vi "BRig_RT__Case_Exp__State_WrongOrTimeout_Pre__v4.vi"(0 "input_dataCurrent":u16[](array[numeric]), 5 "input_WorTO":bool, 7 "input_dataBlock":u16[][](array[numeric]), 9 "input_dataTrial":u16[][](array[numeric]), 11 "input_dataExp":u16[](array[numeric])) -> (1 "output_BTPR":bool, 2 "output_T2R":bool, 3 "output_T2R_or_BTPR":u16, 4 "output_dataCurrent":u16[](array[numeric]), 8 "output_dataBlock":u16[][](array[numeric]), 10 "output_dataTrial":u16[][](array[numeric]), 12 "output_BTPRavg":dbl, 13 "output_T2Ravg":dbl, 14 "output_R(F)_or_L(T)":bool, 15 "output_haveNewAvg":bool)   [LabVIEW 2014]
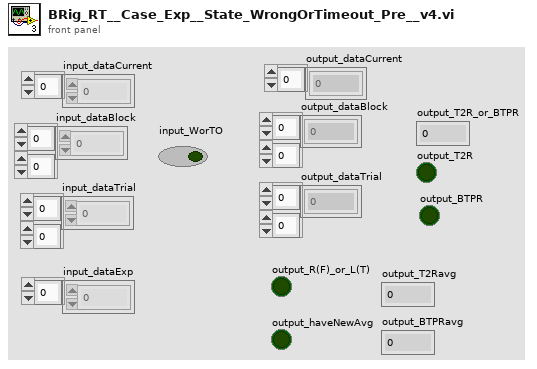
[diagram p1: front panel]
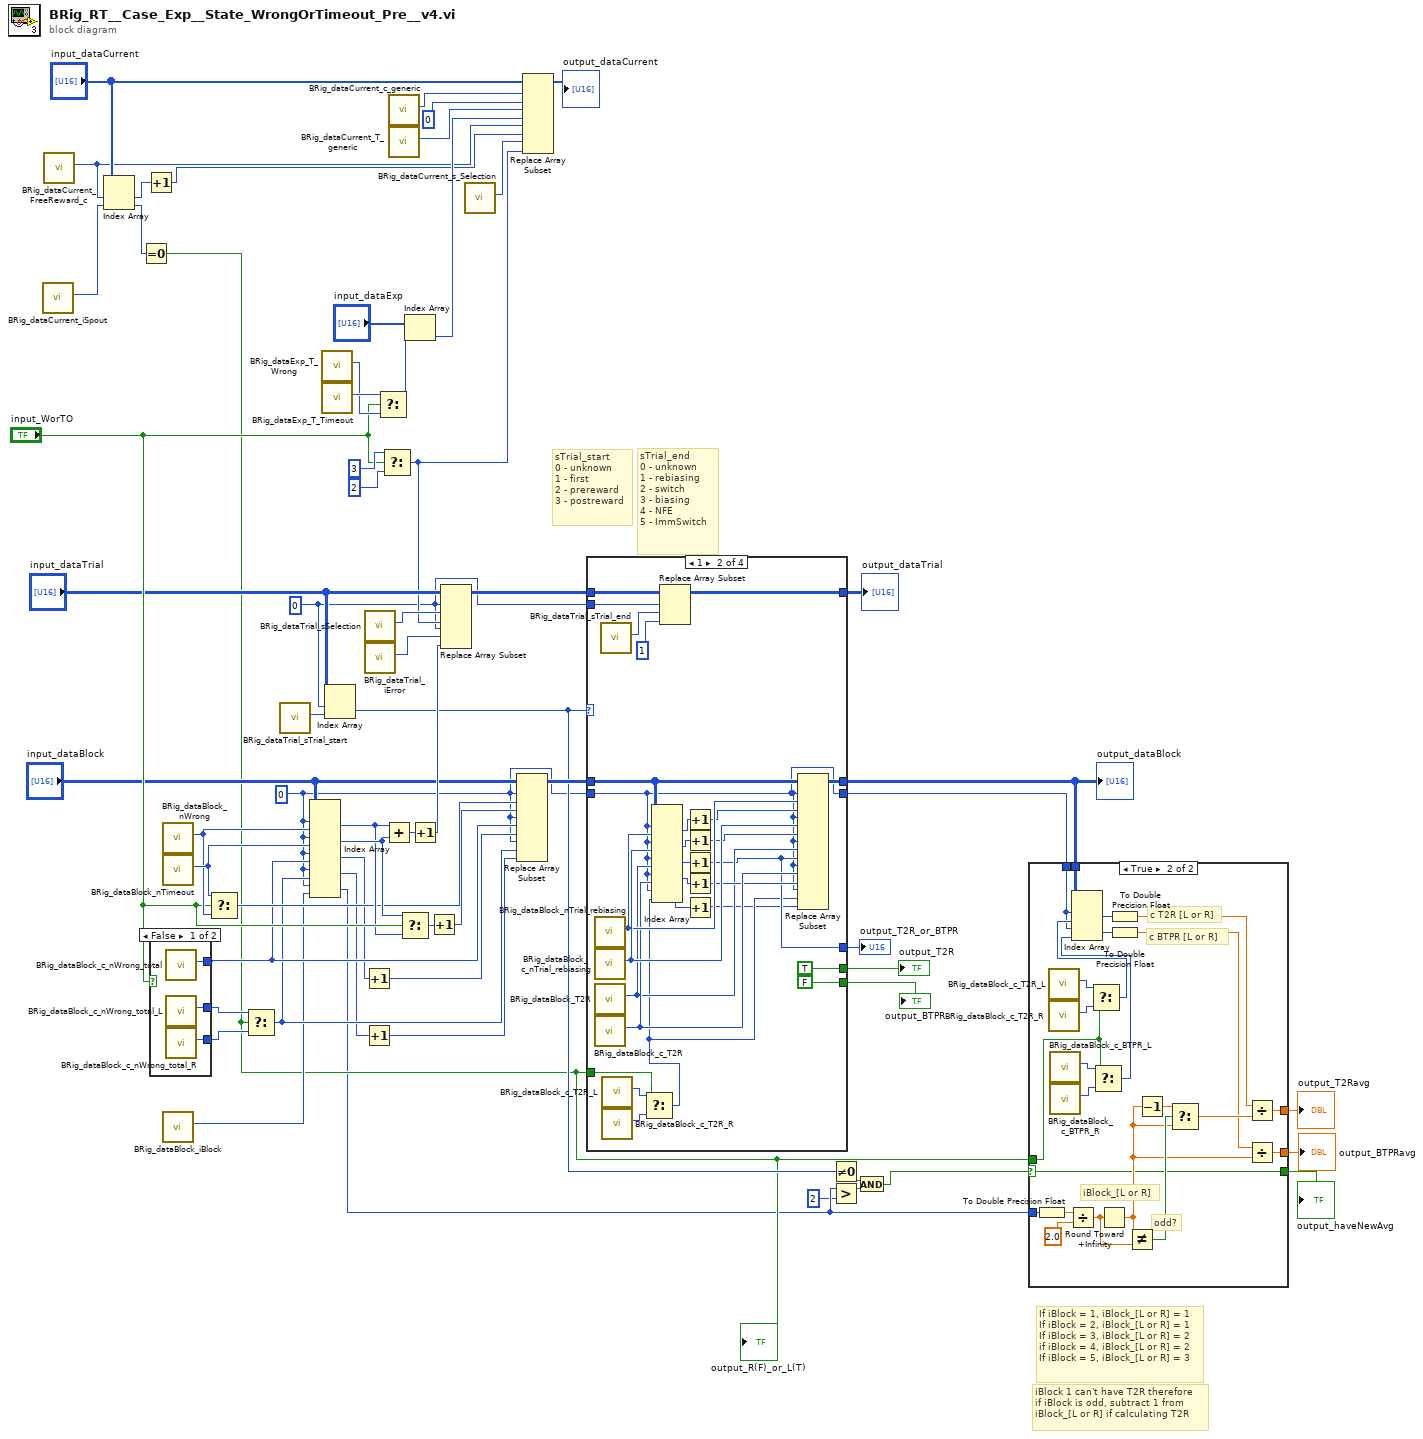
[diagram p0: block diagram]
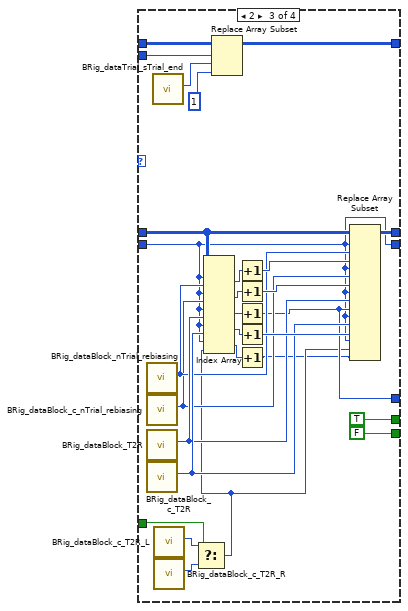
[diagram p4: hidden frame]
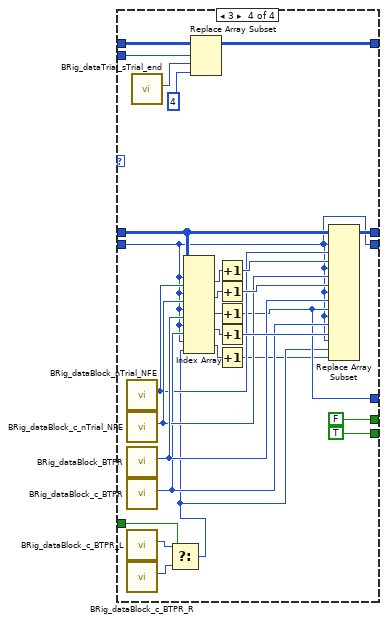
[diagram p5: hidden frame]
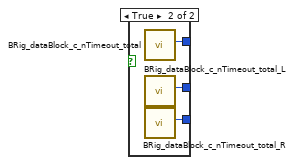
[diagram p6: hidden frame]
diagram:
  w14 = 0
  w15 = 0
  # "iBlock 1 can't have T2R therefore\nif iBlock is odd, subtract 1 from\niBlock_[L or R] if calculating T2R"
  # "If iBlock = 1, iBlock_[L or R] = 1\nIf iBlock = 2, iBlock_[L or R] = 1\nIf iBlock = 3, iBlock_[L or R] = 2\nif iBlock = 4, iBlock_[L or R] = 2\nIf iBlock = 5, iBlock_[L or R] = 3"
  # "sTrial_end\n0 - unknown\n1 - rebiasing\n2 - switch\n3 - biasing\n4 - NFE\n5 - ImmSwitch"
  # "sTrial_start\n0 - unknown\n1 - first\n2 - prereward\n3 - postreward"
  n1 = call "BRig_dataCurrent_iSpout.vi"() -> ("output_iSpout"=w13:i32)  [unwired: 11 in]
  n2 = call "BRig_dataCurrent_FreeReward_c.vi"() -> ("output_FreeReward_c"=w24:i32)  [unwired: 11 in]
  n3 = Index Array(array="input_dataCurrent", index #1=w24, index #2=w13) -> (element #1=w25:u16, element #2=w12:u16)
  n4 = Equal To 0?(x=w12) -> (x = 0?=w11:bool)
  "output_R(F)_or_L(T)" <- w11
  n5 = Increment(x=w25) -> (x+1=w23:u16)
  n6 = case shown="False" "input_WorTO" {
    tunnel: [w66 w69] -> w36
    tunnel: [w65 w68] -> w49
    tunnel: [w64 w67] -> w48
    frame False {
      n7 = call "BRig_dataBlock_c_nWrong_total.vi"() -> ("output_c_nWrong_total"=w66:i32)  [unwired: 11 in]
      n8 = call "BRig_dataBlock_c_nWrong_total_L.vi"() -> ("output_c_nWrong_total_L"=w65:i32)  [unwired: 11 in]
      n9 = call "BRig_dataBlock_c_nWrong_total_R.vi"() -> ("output_c_nWrong_total_R"=w64:i32)  [unwired: 11 in]
    }
    frame True {
      n10 = call "BRig_dataBlock_c_nTimeout_total.vi"() -> ("output_c_nTimeout_total"=w69:i32)  [unwired: 11 in]
      n11 = call "BRig_dataBlock_c_nTimeout_total_L.vi"() -> ("output_c_nTimeout_total_L"=w68:i32)  [unwired: 11 in]
      n12 = call "BRig_dataBlock_c_nTimeout_total_R.vi"() -> ("output_c_nTimeout_total_R"=w67:i32)  [unwired: 11 in]
    }
  }
  n13 = call "BRig_dataBlock_nWrong.vi"() -> ("output_nWrong"=w44:i32)  [unwired: 11 in]
  n14 = call "BRig_dataBlock_nTimeout.vi"() -> ("output_nTimeout"=w45:i32)  [unwired: 11 in]
  n15 = call "BRig_dataBlock_iBlock.vi"() -> ("output_iBlock"=w17:i32)  [unwired: 11 in]
  n16 = Select(t=w45, s="input_WorTO", f=w44) -> (s? t:f=w38:i32)
  n17 = Select(t=w49, s=w11, f=w48) -> (s? t:f=w35:i32)
  n18 = call "BRig_dataTrial_sTrial_start.vi"() -> ("output_sTrial_start"=w30:i32)  [unwired: 11 in]
  n19 = Index Array(array="input_dataBlock", index (row) #1=w14, index (col) #1=w44, index (row) #2=w14, index (col) #2=w45, index (row) #3=w14, index (col) #3=w36, index (row) #4=w14, index (col) #4=w35, index (row) #5=w14, index (col) #5=w17) -> (element #1=w41:u16, element #2=w42:u16, element #3=w34:u16, element #4=w33:u16, element #5=w5:u16)
  n20 = call "BRig_dataExp_T_Wrong.vi"() -> ("output_T_Wrong"=w55:i32)  [unwired: 11 in]
  n21 = call "BRig_dataExp_T_Timeout.vi"() -> ("output_T_Timeout"=w56:i32)  [unwired: 11 in]
  n22 = Index Array(array="input_dataTrial", index (row)=w15, index (col)=w30) -> (element=w16:u16)
  n23 = Increment(x=w34) -> (x+1=w32:u16)
  n24 = Increment(x=w33) -> (x+1=w31:u16)
  n25 = call "BRig_dataTrial_sSelection.vi"() -> ("output_sSelection"=w51:i32)  [unwired: 11 in]
  n26 = call "BRig_dataTrial_iError.vi"() -> ("output_iError"=w50:i32)  [unwired: 11 in]
  n27 = Select(t=w56, s="input_WorTO", f=w55) -> (s? t:f=w57:i32)
  n28 = Select(t=u16 3 ("new element/subarray"), s="input_WorTO", f=u16 2 ("new element/subarray")) -> (s? t:f=w21:u16)
  n29 = Add(x=w41, y=w42) -> (x+y=w47:u16)
  n30 = call "BRig_dataCurrent_c_generic.vi"() -> ("output_count_generic"=w62:i32)  [unwired: 11 in]
  n31 = call "BRig_dataCurrent_T_generic.vi"() -> ("output_T_generic"=w61:i32)  [unwired: 11 in]
  n32 = Select(t=w42, s="input_WorTO", f=w41) -> (s? t:f=w40:u16)
  n33 = Index Array(array="input_dataExp", index=w57) -> (element=w54:u16)
  n34 = Increment(x=w47) -> (x+1=w46:u16)
  n35 = Increment(x=w40) -> (x+1=w37:u16)
  n36 = Replace Array Subset(array="input_dataTrial", new element #1=w21, index (row) #1=w15, index (col) #1=w51, new element #2=w46, index (row) #2=w15, index (col) #2=w50) -> (w28:u16[][])
  n37 = call "BRig_dataCurrent_s_Selection.vi"() -> ("output_s_Selection"=w22:i32)  [unwired: 11 in]
  n38 = Replace Array Subset(array="input_dataBlock", new element #1=w37, index (row) #1=w14, index (col) #1=w38, new element #2=w32, index (row) #2=w14, index (col) #2=w36, new element #3=w31, index (row) #3=w14, index (col) #3=w35) -> (w27:u16[][])
  n39 = Replace Array Subset(array="input_dataCurrent", new element #1=u16 0 ("new element/subarray"), index #1=w62, new element #2=w54, index #2=w61, new element #3=w23, index #3=w24, new element #4=w21, index #4=w22) -> (→"output_dataCurrent":u16[])
  n40 = case shown="1" w16 {
    tunnel: w28 -> [w72 w100 w128 w156]
    tunnel: w15 -> [_ w98 w126 w154]
    tunnel: [w72 w99 w127 w155] -> w26
    tunnel: w27 -> [w71 w89 w112 w144]
    tunnel: [w71 w88 w111 w143] -> w10
    tunnel: w14 -> [w70 w73 w101 w129]
    tunnel: [_ w80 w110 w136] -> w20
    tunnel: [_ TRUE TRUE FALSE] -> w19
    tunnel: [_ FALSE FALSE TRUE] -> w18
    tunnel: w11 -> [_ w79 w103 w135]
    tunnel: [w70 w73 w101 w129] -> w9
    frame 0, Default {
    }
    frame 1 {
      n41 = call "BRig_dataBlock_nTrial_rebiasing.vi"() -> ("output_nTrial_rebiasing"=w94:i32)  [unwired: 11 in]
      n42 = call "BRig_dataBlock_c_nTrial_rebiasing.vi"() -> ("output_c_nTrial_rebiasing"=w95:i32)  [unwired: 11 in]
      n43 = call "BRig_dataBlock_T2R.vi"() -> ("output_T2R"=w83:i32)  [unwired: 11 in]
      n44 = call "BRig_dataBlock_c_T2R.vi"() -> ("output_c_T2R"=w85:i32)  [unwired: 11 in]
      n45 = call "BRig_dataTrial_sTrial_end.vi"() -> ("output_sTrial_end"=w97:i32)  [unwired: 11 in]
      n46 = call "BRig_dataBlock_c_T2R_L.vi"() -> ("output_c_T2R_L"=w78:i32)  [unwired: 11 in]
      n47 = call "BRig_dataBlock_c_T2R_R.vi"() -> ("output_c_T2R_R"=w77:i32)  [unwired: 11 in]
      n48 = Select(t=w78, s=w79, f=w77) -> (s? t:f=w75:i32)
      n49 = Index Array(array=w89, index (row) #1=w73, index (col) #1=w94, index (row) #2=w73, index (col) #2=w95, index (row) #3=w73, index (col) #3=w83, index (row) #4=w73, index (col) #4=w85, index (row) #5=w73, index (col) #5=w75) -> (element #1=w93:u16, element #2=w91:u16, element #3=w87:u16, element #4=w86:u16, element #5=w76:u16)
      n50 = Replace Array Subset(array=w100, new element=u16 1 ("new element/subarray"), index (row)=w98, index (col)=w97) -> (w99:u16[][])
      n51 = Increment(x=w93) -> (x+1=w92:u16)
      n52 = Increment(x=w91) -> (x+1=w90:u16)
      n53 = Increment(x=w87) -> (x+1=w80:u16)
      n54 = Increment(x=w86) -> (x+1=w84:u16)
      n55 = Increment(x=w76) -> (x+1=w74:u16)
      n56 = Replace Array Subset(array=w89, new element #1=w92, index (row) #1=w73, index (col) #1=w94, new element #2=w90, index (row) #2=w73, index (col) #2=w95, new element #3=w80, index (row) #3=w73, index (col) #3=w83, new element #4=w84, index (row) #4=w73, index (col) #4=w85, new element #5=w74, index (row) #5=w73, index (col) #5=w75) -> (w88:u16[][])
    }
    frame 2 {
      n57 = call "BRig_dataBlock_nTrial_rebiasing.vi"() -> ("output_nTrial_rebiasing"=w114:i32)  [unwired: 11 in]
      n58 = call "BRig_dataBlock_c_nTrial_rebiasing.vi"() -> ("output_c_nTrial_rebiasing"=w113:i32)  [unwired: 11 in]
      n59 = call "BRig_dataBlock_T2R.vi"() -> ("output_T2R"=w121:i32)  [unwired: 11 in]
      n60 = call "BRig_dataBlock_c_T2R.vi"() -> ("output_c_T2R"=w122:i32)  [unwired: 11 in]
      n61 = call "BRig_dataTrial_sTrial_end.vi"() -> ("output_sTrial_end"=w125:i32)  [unwired: 11 in]
      n62 = call "BRig_dataBlock_c_T2R_L.vi"() -> ("output_c_T2R_L"=w107:i32)  [unwired: 11 in]
      n63 = call "BRig_dataBlock_c_T2R_R.vi"() -> ("output_c_T2R_R"=w106:i32)  [unwired: 11 in]
      n64 = Select(t=w107, s=w103, f=w106) -> (s? t:f=w104:i32)
      n65 = Index Array(array=w112, index (row) #1=w101, index (col) #1=w114, index (row) #2=w101, index (col) #2=w113, index (row) #3=w101, index (col) #3=w121, index (row) #4=w101, index (col) #4=w122, index (row) #5=w101, index (col) #5=w104) -> (element #1=w115:u16, element #2=w117:u16, element #3=w119:u16, element #4=w120:u16, element #5=w105:u16)
      n66 = Replace Array Subset(array=w128, new element=u16 1 ("new element/subarray"), index (row)=w126, index (col)=w125) -> (w127:u16[][])
      n67 = Increment(x=w115) -> (x+1=w116:u16)
      n68 = Increment(x=w117) -> (x+1=w118:u16)
      n69 = Increment(x=w119) -> (x+1=w110:u16)
      n70 = Increment(x=w120) -> (x+1=w123:u16)
      n71 = Increment(x=w105) -> (x+1=w102:u16)
      n72 = Replace Array Subset(array=w112, new element #1=w116, index (row) #1=w101, index (col) #1=w114, new element #2=w118, index (row) #2=w101, index (col) #2=w113, new element #3=w110, index (row) #3=w101, index (col) #3=w121, new element #4=w123, index (row) #4=w101, index (col) #4=w122, new element #5=w102, index (row) #5=w101, index (col) #5=w104) -> (w111:u16[][])
    }
    frame 3 {
      n73 = call "BRig_dataBlock_nTrial_NFE.vi"() -> ("output_nTrial_NFE"=w139:i32)  [unwired: 11 in]
      n74 = call "BRig_dataBlock_c_nTrial_NFE.vi"() -> ("output_c_nTrial_NFE"=w141:i32)  [unwired: 11 in]
      n75 = call "BRig_dataBlock_BTPR.vi"() -> ("output_BTPR"=w142:i32)  [unwired: 11 in]
      n76 = call "BRig_dataBlock_c_BTPR.vi"() -> ("output_c_BTPR"=w140:i32)  [unwired: 11 in]
      n77 = call "BRig_dataBlock_c_BTPR_L.vi"() -> ("output_c_BTPR_L"=w134:i32)  [unwired: 11 in]
      n78 = call "BRig_dataBlock_c_BTPR_R.vi"() -> ("output_c_BTPR_R"=w133:i32)  [unwired: 11 in]
      n79 = call "BRig_dataTrial_sTrial_end.vi"() -> ("output_sTrial_end"=w153:i32)  [unwired: 11 in]
      n80 = Select(t=w134, s=w135, f=w133) -> (s? t:f=w131:i32)
      n81 = Index Array(array=w144, index (row) #1=w129, index (col) #1=w139, index (row) #2=w129, index (col) #2=w141, index (row) #3=w129, index (col) #3=w142, index (row) #4=w129, index (col) #4=w140, index (row) #5=w129, index (col) #5=w131) -> (element #1=w145:u16, element #2=w147:u16, element #3=w149:u16, element #4=w150:u16, element #5=w132:u16)
      n82 = Replace Array Subset(array=w156, new element=u16 4 ("new element/subarray"), index (row)=w154, index (col)=w153) -> (w155:u16[][])
      n83 = Increment(x=w145) -> (x+1=w146:u16)
      n84 = Increment(x=w147) -> (x+1=w148:u16)
      n85 = Increment(x=w149) -> (x+1=w136:u16)
      n86 = Increment(x=w150) -> (x+1=w151:u16)
      n87 = Increment(x=w132) -> (x+1=w130:u16)
      n88 = Replace Array Subset(array=w144, new element #1=w146, index (row) #1=w129, index (col) #1=w139, new element #2=w148, index (row) #2=w129, index (col) #2=w141, new element #3=w136, index (row) #3=w129, index (col) #3=w142, new element #4=w151, index (row) #4=w129, index (col) #4=w140, new element #5=w130, index (row) #5=w129, index (col) #5=w131) -> (w143:u16[][])
    }
  }
  "output_dataBlock" <- w10
  "output_dataTrial" <- w26
  "output_T2R_or_BTPR" <- w20
  "output_T2R" <- w19
  "output_BTPR" <- w18
  n89 = Not Equal To 0?(x=w16) -> (x != 0?=w2:bool)
  n90 = Greater?(x=w5, y=u16 2) -> (0:w3:bool)
  n91 = And(x=w2, y=w3) -> (x .and. y?=w1:bool)
  n92 = case shown="True" w1 {
    selector: w1 -> [_ w157]
    tunnel: w11 -> [_ w172]
    tunnel: w10 -> [_ w175]
    tunnel: w9 -> [_ w174]
    tunnel: w5 -> [_ w168]
    tunnel: [_ w159] -> w8
    tunnel: [_ w158] -> w7
    tunnel: [_ w157] -> w6
    frame False {
    }
    frame True {
      # "c BTPR [L or R]"
      # "c T2R [L or R]"
      # "odd?"
      # "iBlock_[L or R]"
      n93 = To Double Precision Float(number=w168) -> (double precision float=w171:dbl)
      n94 = call "BRig_dataBlock_c_T2R_L.vi"() -> ("output_c_T2R_L"=w179:i32)  [unwired: 11 in]
      n95 = call "BRig_dataBlock_c_T2R_R.vi"() -> ("output_c_T2R_R"=w180:i32)  [unwired: 11 in]
      n96 = call "BRig_dataBlock_c_BTPR_L.vi"() -> ("output_c_BTPR_L"=w177:i32)  [unwired: 11 in]
      n97 = call "BRig_dataBlock_c_BTPR_R.vi"() -> ("output_c_BTPR_R"=w178:i32)  [unwired: 11 in]
      n98 = Divide(x=w171, y=2.0) -> (x/y=w169:dbl)
      n99 = Select(t=w179, s=w172, f=w180) -> (s? t:f=w176:i32)
      n100 = Select(t=w177, s=w172, f=w178) -> (s? t:f=w173:i32)
      n101 = Index Array(array=w175, index (row) #1=w174, index (col) #1=w176, index (row) #2=w174, index (col) #2=w173) -> (element #1=w163:u16, element #2=w164:u16)
      n102 = Round Toward +Infinity(x=w169) -> (ceil(x): smallest int >= x=w162:dbl)
      n103 = To Double Precision Float(number=w163) -> (double precision float=w161:dbl)
      n104 = To Double Precision Float(number=w164) -> (double precision float=w160:dbl)
      n105 = Not Equal?(x=w162, y=w169) -> (x != y?=w166:bool)
      n106 = Decrement(x=w162) -> (x-1=w167:dbl)
      n107 = Select(t=w167, s=w166, f=w162) -> (s? t:f=w165:dbl)
      n108 = Divide(x=w161, y=w165) -> (x/y=w159:dbl)
      n109 = Divide(x=w160, y=w162) -> (x/y=w158:dbl)
    }
  }
  "output_T2Ravg" <- w8
  "output_BTPRavg" <- w7
  "output_haveNewAvg" <- w6
